vi "DDTProbe.vi"(1 "Dynamic data in":dynamicdata(waveform)) -> (0 "Stop?":bool)   [LabVIEW 2020]
doc: "Displays the attributes for each waveform and graphs the data."
panel:
  in  "x dim Y":string="f"
  in  "Time":string="Time (sec)"
  in  "Freq":string="Frequency (Hz)"
  in  "x dim X":string="t"
  in  "Rel":string="Relative"
  in  "Abs":string="Absolute"
  in  "Tab Control":enum32{"Data   ", "Graph     "}(tab)
  out "?":T1(array[cluster]) {"Timestamp" format="%<%X\n%x>T"; "Start timestamp" format="%<%X\n%x>T"}
  out "Waveform Graph":dynamicdata(graph)
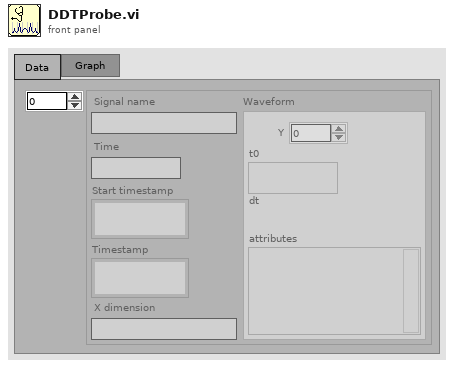
[diagram p1: front panel]
types:
  T1 = cluster{"Waveform":waveform(dbl), "Signal name":string, "Time":string, "Start timestamp":timestamp, "Timestamp":timestamp, "X dimension":string}[]
  T2 = typedef "ex_WaveformAttribs.ctl" = cluster{"Start Timestamp":timestamp, "Timestamp":timestamp, "Relative Time?":bool, "X Dimension":string, "Signal Name":string}
  T3 = cluster{"waveform":waveform(dbl), "Signal Name":string, "Rel":string, "Start Timestamp":timestamp, "Timestamp":timestamp, "Time":string}
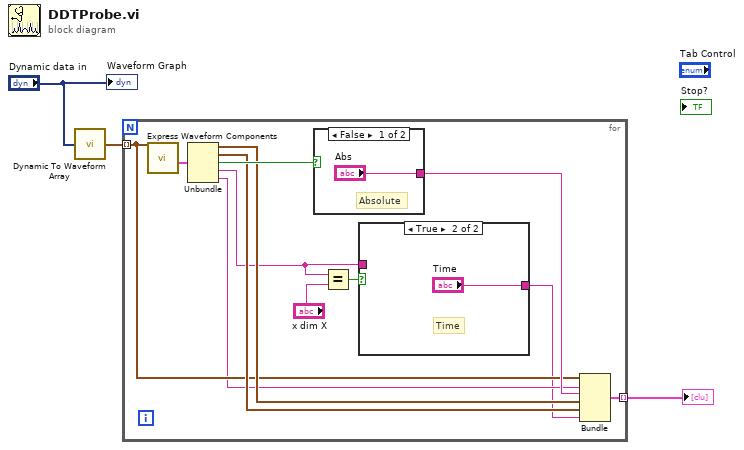
[diagram p0: block diagram]
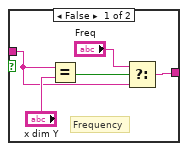
[diagram p2: hidden frame]
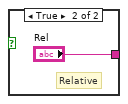
[diagram p3: hidden frame]
diagram:
  n1 = call <vilib>:"Dynamic To Waveform Array.vi"("Input"="Dynamic data in") -> ("Output"=w2:waveform(dbl)[])  [unwired: 4 in]
  n2 = for {
    tunnel: w2 -> [w9] mode=indexing
    tunnel: [w10] -> w1 mode=indexing
    n3 = call <vilib>:"Express Waveform Components.vi"("Waveform"=w9) -> ("Express Waveform Attributes"=w15:T2)  [unwired: 7 in, 3 out]
    n4 = Unbundle(w15) -> ("Start Timestamp"=w12:timestamp, "Timestamp"=w11:timestamp, "Relative Time?"=w14:bool, "X Dimension"=w4:string, "Signal Name"=w8:string)
    n5 = case shown="False" w14 {
      tunnel: ["Abs" "Rel"] -> w13
      frame False {
        # "Absolute"
      }
      frame True {
        # "Relative"
      }
    }
    n6 = Equal?(x=w4, y="x dim X") -> (x = y?=w6:bool)
    n7 = case shown="True" w6 {
      tunnel: [w17 "Time"] -> w5
      tunnel: w4 -> [w16 _]
      frame False {
        # "Frequency"
        n8 = Equal?(x=w16, y="x dim Y") -> (x = y?=w19:bool)
        n9 = Select(t="Freq", s=w19, f=w16) -> (s? t:f=w17:string)
      }
      frame True {
        # "Time"
      }
    }
    n10 = Bundle("waveform"=w9, "Signal Name"=w8, "Rel"=w13, "Start Timestamp"=w12, "Timestamp"=w11, "Time"=w5) -> (w10:T3)  [unwired: 1 in]
  }
  "?" <- w1
  "Waveform Graph" <- "Dynamic data in"
